vi "DAQmx INIT.vi"(8 "error in":errorcluster, 10 "task name":string="Signal", 11 "DAQmxChannel":T1) -> (0 "error out":errorcluster, 3 "task out":refnum<k21>)   [LabVIEW 2020]
uses:
  <vilib>/DAQmx/configure/timing.llb/DAQmx Timing (Sample Clock).vi
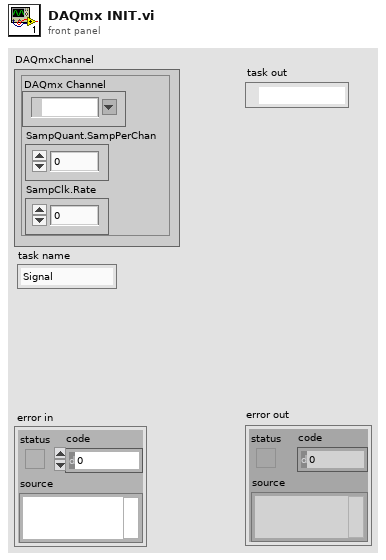
[diagram p1: front panel]
types:
  T1 = cluster{"SampClk.Rate":dbl, "SampQuant.SampPerChan":i32, "DAQmx Channel":refnum<k21>}
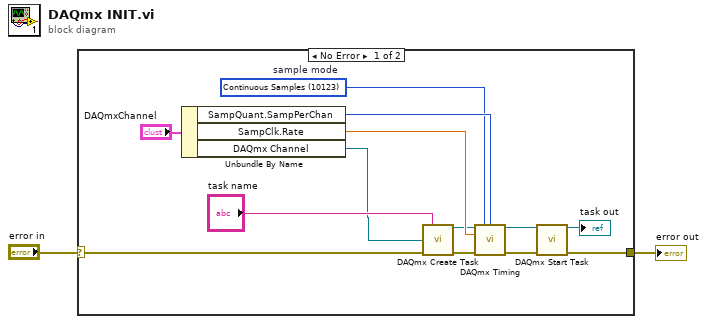
[diagram p0: block diagram]
diagram:
  n1 = case shown="No Error" "error in" {
    selector: "error in" -> [w11 w16]
    tunnel: [w10 w16] -> w2
    frame No Error {
      w13 = 10123 items=["Finite Samples"=10178, "Continuous Samples"=10123, "Hardware Timed Single Point"=12522]  # sample mode
      n2 = Unbundle By Name("DAQmxChannel") -> ("SampQuant.SampPerChan"=w15:i32, "SampClk.Rate"=w14:dbl, "DAQmx Channel"=w3:refnum<k21>)
      n3 = call <vilib>:"DAQmx Create Task.vi"("new task name"="task name", "global virtual channels"=w3, "error in"=w11) -> ("task out"=w5:refnum<k21>, "error out"=w4:errorcluster)  [unwired: 11 in]
      n4 = call-poly <vilib>:"DAQmx Timing.vi"("task/channels in"=w5, "sample mode"=w13, "samples per channel"=w15, "rate"=w14, "error in"=w4) -> ("task out"=w9:refnum<k21>, "error out"=w12:errorcluster)  [unwired: 9 in]
      n5 = call <vilib>:"DAQmx Start Task.vi"("task/channels in"=w9, "error in"=w12) -> ("task out"=→"task out":refnum<k21>, "error out"=w10:errorcluster)  [unwired: 12 in]
    }
    frame Error {
    }
  }
  "error out" <- w2
